vi "G1G2Converter_Tool_GenerateExcludeClassesIni.vi"() -> ()   [LabVIEW 2009]
panel:
  out "error out":errorcluster
  in  "Folder Path":path
  in  "Treat LLBs as Folders?":bool=TRUE
  # "Generates the ExcludeClasses.ini file in the specified folder. All folders will be added."
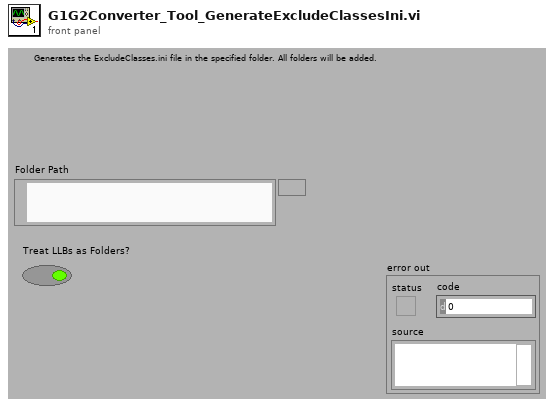
[diagram p1: front panel]
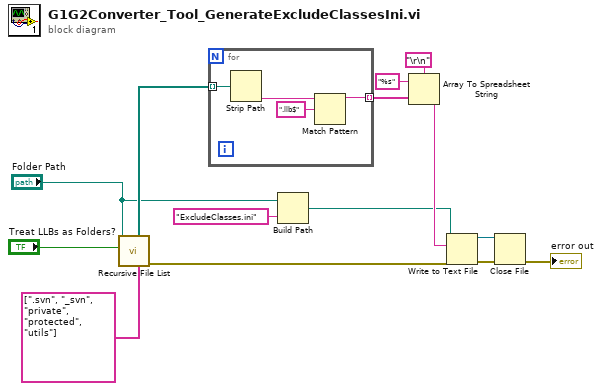
[diagram p0: block diagram]
diagram:
  n1 = call <vilib>:"Recursive File List.vi"("Folders to Exclude"=string[] [".svn", "_svn", "private", "protected", "utils"], "Treat LLBs as Folders?"="Treat LLBs as Folders?", "Folder Path"="Folder Path") -> ("error out"=w11:errorcluster, "All Folders"=w12:path[])  [unwired: 4 in, 3 out]
  n2 = for {
    tunnel: w12 -> [w18] mode=indexing
    tunnel: [w15] -> w10 mode=indexing
    n3 = Strip Path(path=w18) -> (name=w17:string)  [unwired: 1 out]
    n4 = Match Pattern(string=w17, regular expression=".llb$") -> (before substring=w15:string)  [unwired: 1 in, 3 out]
  }
  n5 = Build Path(base path="Folder Path", name or relative path="ExcludeClasses.ini") -> (appended path=w4:path)
  n6 = Array To Spreadsheet String(delimiter (Tab)="\r\n", array=w10, 3:"%s" ("format string")) -> (spreadsheet string=w7:string)
  n7 = Write to Text File(file (use dialog)=w4, text=w7, error in=w11) -> (refnum out=w2:refnum<file>, error out=w3:errorcluster)  [unwired: 1 in, 1 out]
  n8 = Close File(refnum=w2, error in=w3) -> (error out=→"error out":errorcluster)  [unwired: 1 out]
